vi "3458A Get Max Aperture for Sampling Rate.vi"(1 "fs [Hz]":dbl format="%#_6p") -> (0 "ta_max [s]":dbl format="%#_6p")   [LabVIEW 2018, in "3458A Virtual Digitizer.lvlib" / "3458A Digitizing Low Levels.lvlib"]
doc: "Gets maximum aperture time for given sampling rate for DCV mode."
uses:
  3458A Digitizing Low Levels.lvlib
panel:
  out "XY Graph":cluster{dbl[], dbl[]}(graph)
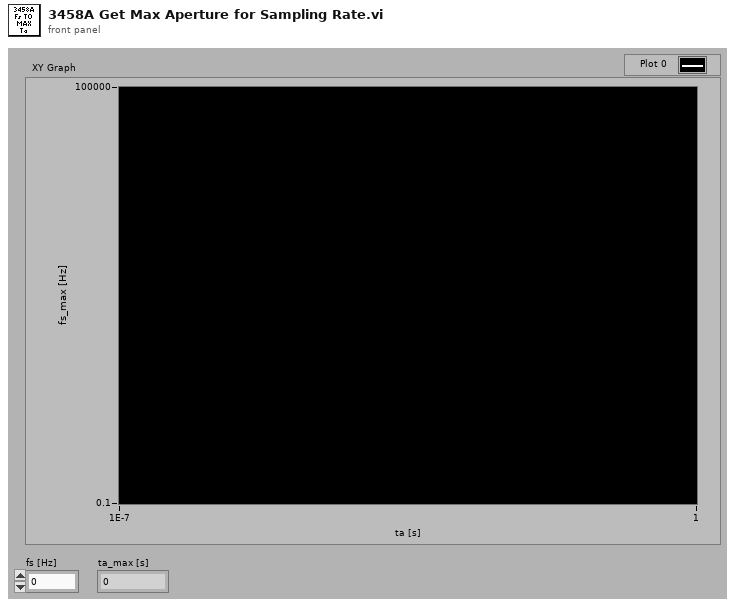
[diagram p1: front panel]
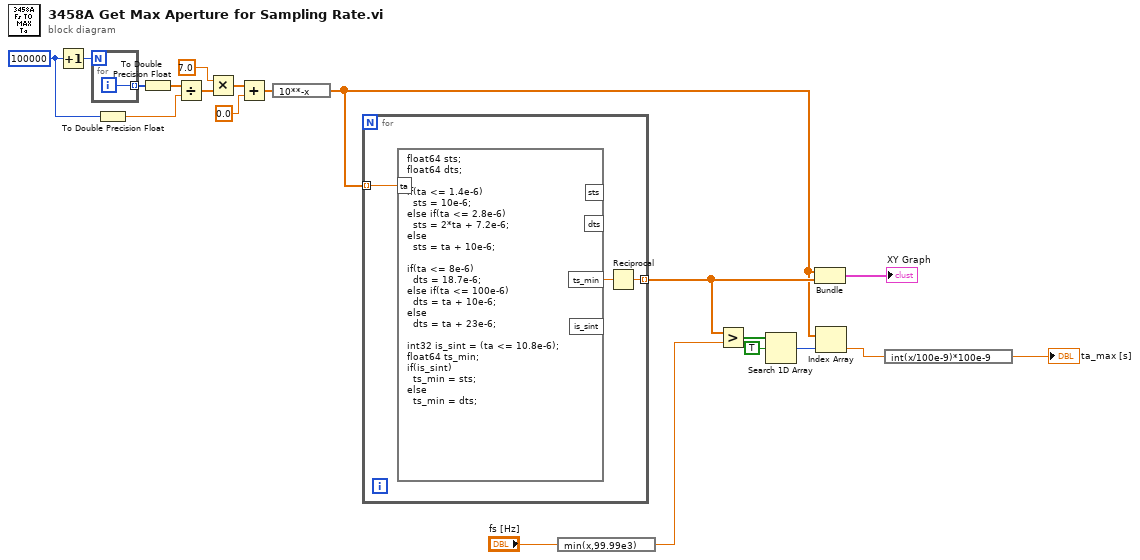
[diagram p0: block diagram]
diagram:
  w17 = 100000
  n1 = Increment(x=w17) -> (x+1=w19:i32)
  n2 = for {
    N: w19 -> [_]
    tunnel: [w21] -> w20 mode=indexing
    i -> [w21]
  }
  n3 = To Double Precision Float(number=w17) -> (double precision float=w16:dbl)
  n4 = To Double Precision Float(number=w20) -> (double precision float=w18:dbl[])
  n5 = Divide(x=w18, y=w16) -> (x/y=w15:dbl[])
  n6 = Multiply(x=7.0, y=w15) -> (x*y=w13:dbl[])
  n7 = Add(x=w13, y=0.0) -> (x+y=w11:dbl[])
  n8 = expression code="10**-x"(w11) -> (w5:dbl[])
  n9 = for {
    tunnel: w5 -> [w23] mode=indexing
    tunnel: [w22] -> w10 mode=indexing
    n10 = formula code="float64 sts;\nfloat64 dts;\n\nif(ta <= 1.4e-6)\n  sts = 10e-6;\nelse if(ta <= 2.8e-6)\n  sts = 2*ta + 7.2e-6;\nelse\n  sts = ta + 10e-6;\n\nif(ta <= 8e-6)\n  dts = 18.7e-6;\nelse if(ta <= 100e-6)\n  dts = ta + 10e-6;\nelse\n  dts = ta + 23e-6;\n\nint32 is_sint = (ta <= 10.8e-6);\nfloat64 ts_min;\nif(is_sint)\n  ts_min = sts;\nelse\n  ts_min = dts;"("ta"=w23) -> ("ts_min"=w24:dbl)  [unwired: 3 out]
    n11 = Reciprocal(x=w24) -> (1/x=w22:dbl)
  }
  n12 = expression code="min(x,99.99e3)"("fs [Hz]") -> (w1:dbl)
  n13 = Greater?(x=w10, y=w1) -> (0:w8:bool[])
  n14 = Search 1D Array(1D array=w8, element=TRUE) -> (index of element=w6:i32)  [unwired: 1 in]
  n15 = Bundle(w5, w10) -> (→"XY Graph":cluster{dbl[], dbl[]})  [unwired: 1 in]
  n16 = Index Array(array=w5, index=w6) -> (element=w4:dbl)
  n17 = expression code="int(x/100e-9)*100e-9"(w4) -> (→"ta_max [s]":dbl)
